vi "Set Caption.vi"(8 "error in":errorcluster, 10 "Caption":string, 11 "Check Box in":refnum<class "Check Box.lvclass">) -> (0 "error out":errorcluster, 3 "Check Box out":refnum<class "Check Box.lvclass">)   [LabVIEW 2024, in "SourceGrid.lvlib" / "Check Box.lvclass"]
uses:
  Check Box.lvclass
  D:/git/Sourcegrid-LabVIEW/dll/SourceGrid.dll
  dll/SourceGrid.dll
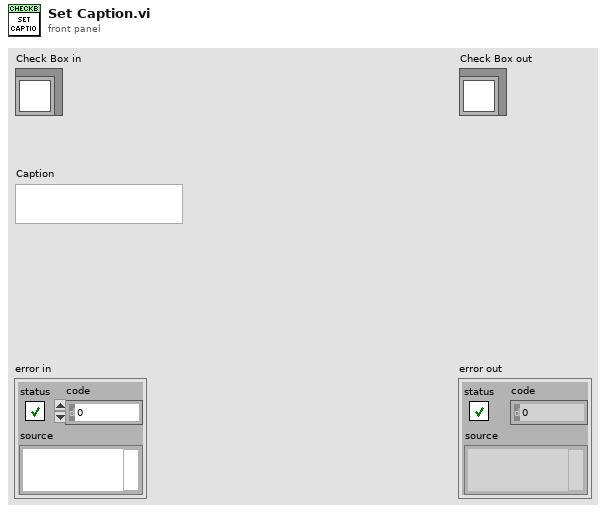
[diagram p1: front panel]
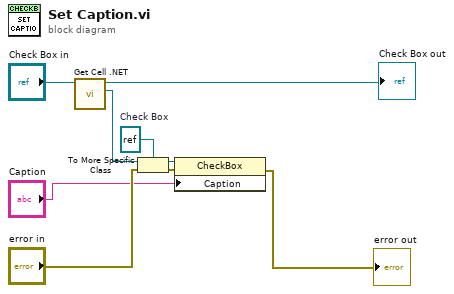
[diagram p0: block diagram]
diagram:
  w4 = refnum<k24> refnum  # Check Box
  n1 = call-dynamic "Get Cell .NET.vi"("Cell in"="Check Box in") -> ("Cell .NET"=w7:refnum<k24>, "Cell out"=→"Check Box out":refnum<class "Check Box.lvclass">)  [unwired: 9 in]
  n2 = To More Specific Class(target class=w4, reference=w7, error in="error in") -> (specific class reference=w5:refnum<k24>, error out=w3:errorcluster)
  n3 = property class="CheckBox"(reference=w5, error in=w3, "Caption"="Caption") -> (error out=→"error out":errorcluster)  [unwired: 1 out]
